vi "setTitle.vi"(7 "Offset":cluster{"horizontal":dbl, "vertical":dbl}, 8 "Set?":bool=TRUE, 9 "Title":string, 11 "String in":string) -> (2 "command":string, 3 "String out":string)   [LabVIEW 2013]
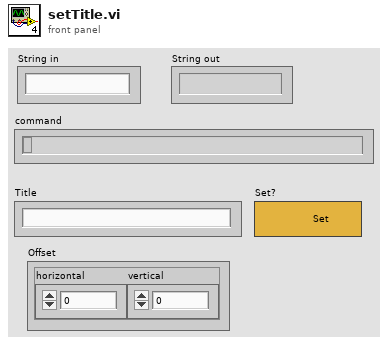
[diagram p1: front panel]
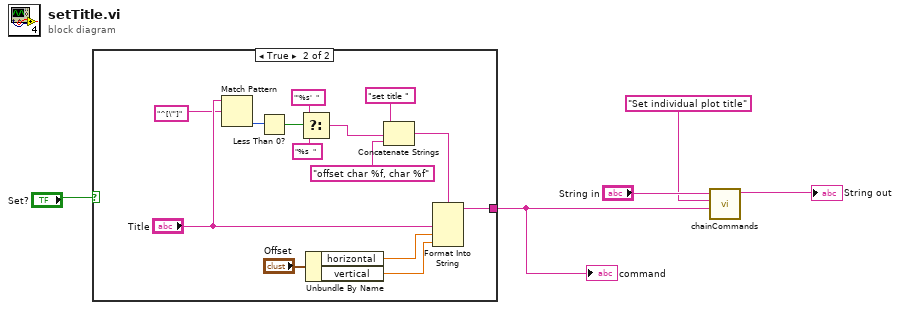
[diagram p0: block diagram]
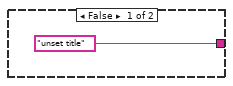
[diagram p2: hidden frame]
diagram:
  n1 = case shown="True" "Set?" {
    tunnel: ["unset title" w20] -> w4
    frame False {
    }
    frame True {
      n2 = Match Pattern(string="Title", regular expression="^[\"']") -> (offset past match=w16:i32)  [unwired: 1 in, 3 out]
      n3 = Less Than 0?(x=w16) -> (x < 0?=w15:bool)
      n4 = Select(t="'%s'  " ("format string"), s=w15, f="%s  " ("format string")) -> (s? t:f=w10:string)
      n5 = Unbundle By Name("Offset") -> ("horizontal"=w18:dbl, "vertical"=w17:dbl)
      n6 = Concatenate Strings("set title " ("format string"), w10, "offset char %f, char %f" ("format string")) -> (w7:string)
      n7 = Format Into String(format string=w7, "Title", w18, w17) -> (resulting string=w20:string)  [unwired: 2 in, 1 out]
    }
  }
  "command" <- w4
  n8 = call "chainCommands.vi"("Command"=w4, "Comments"="Set individual plot title", "StringIn"="String in") -> ("StringOut"=→"String out":string)  [unwired: 8 in]
